vi "FillContents.vi"(9 "display in":picture, 11 "Cell in":refnum<class "Cell.lvclass">) -> (1 "display out":picture, 3 "Cell out":refnum<class "Cell.lvclass">)   [LabVIEW 2021, in "Cell.lvclass"]
uses:
  Cell.lvclass
  Cell.lvclass/Cell.ctl
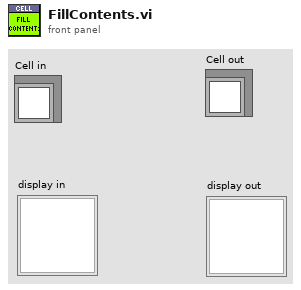
[diagram p1: front panel]
types:
  T1 = cluster{"left":i16, "top":i16, "right":i16, "bottom":i16}
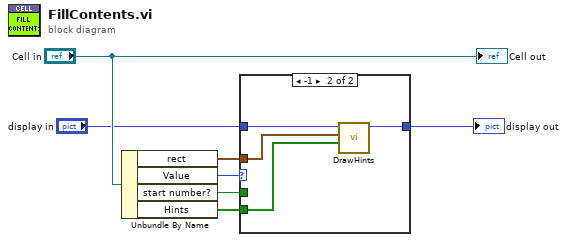
[diagram p0: block diagram]
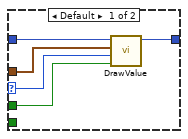
[diagram p2: hidden frame]
diagram:
  n1 = Unbundle By Name("Cell in") -> ("rect"=w3:T1, "Value"=w6:i8, "start number?"=w2:bool, "Hints"=w1:bool[])
  n2 = case shown="-1" w6 {
    selector: w6 -> [w10 _]
    tunnel: "display in" -> [w12 w16]
    tunnel: [w11 w15] -> w4
    tunnel: w3 -> [w9 w14]
    tunnel: w2 -> [w8 _]
    tunnel: w1 -> [_ w13]
    frame Default {
      n3 = call "DrawValue.vi"("start number?"=w8, "Value"=w10, "rect"=w9, "picture in"=w12) -> ("picture out"=w11:picture)  [unwired: 7 in]
    }
    frame -1 {
      n4 = call "DrawHints.vi"("Hints"=w13, "rect"=w14, "picture in"=w16) -> ("picture out"=w15:picture)  [unwired: 8 in]
    }
  }
  "display out" <- w4
  "Cell out" <- "Cell in"
